vi "Read Running VI reference.vi"(8 "error in (no error)":errorcluster, 11 "Fiber Auto Collimation panel in":refnum<class "Fiber Auto Collimation panel.lvclass">) -> (0 "error out":errorcluster, 2 "Running VI reference":refnum<vi>, 3 "Fiber Auto Collimation panel out":refnum<class "Fiber Auto Collimation panel.lvclass">)   [LabVIEW 2018, in "Fiber Auto Collimation panel.lvclass"]
doc: "Reads a reference to the running VI of this Panel class.\n\nNote that this is a member of class data, and not an \"obtain global\" function of any kind. If this reference is read from a class coming from the \"Check panel run status\" VI that says it is running, it is probably always a real and current reference. If it comes from anywhere else, it might have been never written to, or a reference to a panel that was open but is now closed.\n\nNote: The Apex VI will never return a reference from this."
uses:
  Fiber Auto Collimation panel.lvclass
  Fiber Auto Collimation panel.lvclass/Fiber Auto Collimation panel.ctl
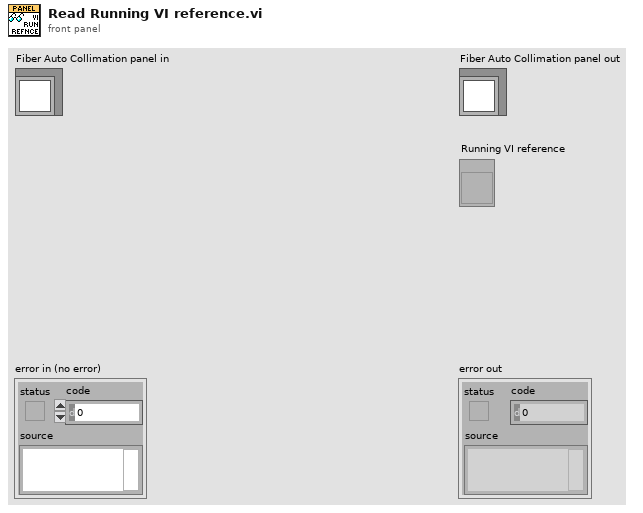
[diagram p1: front panel]
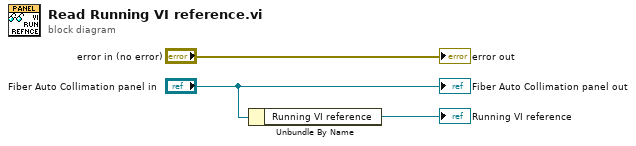
[diagram p0: block diagram]
diagram:
  n1 = Unbundle By Name("Fiber Auto Collimation panel in") -> ("Running VI reference"=→"Running VI reference":refnum<vi>)
  "error out" <- "error in (no error)"
  "Fiber Auto Collimation panel out" <- "Fiber Auto Collimation panel in"
